vi "Interleave 2D array.vi"(1 "2D":dbl[][](array[numeric]) format="%.2f") -> (0 "1D":dbl[](array[numeric]) format="%.2f")   [LabVIEW 2010]
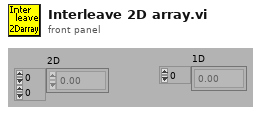
[diagram p1: front panel]
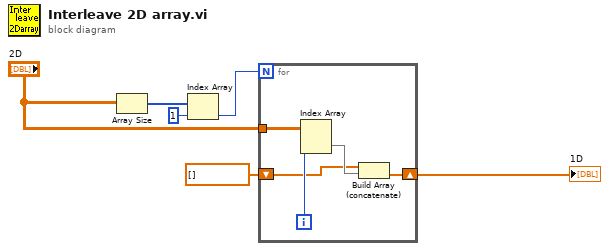
[diagram p0: block diagram]
diagram:
  n1 = Array Size(array="2D") -> (size(s)=w1:i32[])
  n2 = Index Array(array=w1, index=1 ("Index")) -> (element=w3:i32)
  n3 = for {
    N: w3 -> [_]
    tunnel: "2D" -> [w10]
    shift-right: [w11] -> w4
    shift-left: dbl[] [] -> [w7]
    i -> [w9]
    n4 = Index Array(array=w10, index (col)=w9) -> (element=w8:dbl[])  [unwired: 1 in]
    n5 = Build Array (concatenate)(w7, w8) -> (w11:dbl[])
  }
  "1D" <- w4
